vi "Write session and device.vi"(8 "error in (no error)":errorcluster, 9 "SLSC Device":refnum<k21>, 10 "SLSC Session in":refnum<class "SLSC Interface.lvclass">, 11 "SLSC Switch in":refnum<class "SLSC Switch.lvclass">) -> (0 "error out":errorcluster, 3 "SLSC Switch out":refnum<class "SLSC Switch.lvclass">)   [LabVIEW 2015, in "SLSC Switch.lvlib" / "SLSC Switch.lvclass"]
uses:
  SLSC Switch.lvclass
  <vilib>/National Instruments/SLSC Local or Remote Interface/SLSC Interface Class/SLSC Interface.lvclass
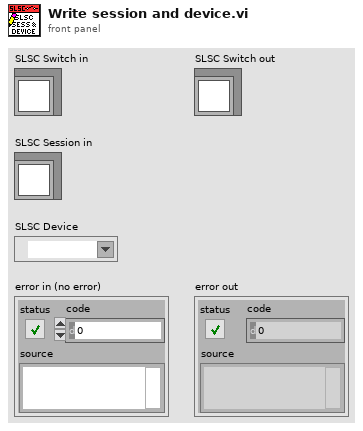
[diagram p1: front panel]
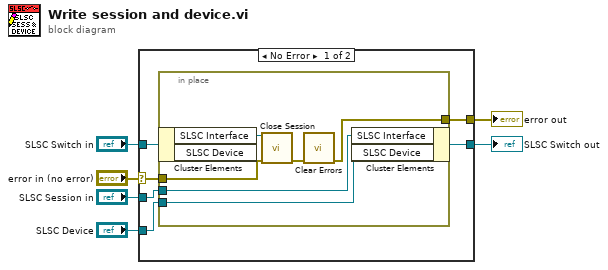
[diagram p0: block diagram]
diagram:
  n1 = case shown="No Error" "error in (no error)" {
    selector: "error in (no error)" -> [w10 w19]
    tunnel: "SLSC Switch in" -> [w12 w20]
    tunnel: [w11 w20] -> w5
    tunnel: [w9 w19] -> w3
    tunnel: "SLSC Device" -> [w8 _]
    tunnel: "SLSC Session in" -> [w7 _]
    frame No Error {
      n2 = in-place {
        in-place-border: w10 -> [w14]
        in-place-border: [w18] -> w9
        in-place-border: w8 -> [w17]
        in-place-border: w7 -> [w16]
        n3 = in-place-cluster #1(w12) -> ("SLSC Interface"=w15:refnum<class "SLSC Interface.lvclass">)  [unwired: 1 out]
        n4 = call-dynamic "Close Session.vi"("SLSC Interface in"=w15, "error in (no error)"=w14) -> ("error out"=w13:errorcluster)  [unwired: 13 in]
        n5 = call <vilib>:"Clear Errors.vi"("error in (no error)"=w13) -> ("error out"=w18:errorcluster)  [unwired: 5 in, 1 out]
        n6 = in-place-cluster #1("SLSC Interface"=w16, "SLSC Device"=w17) -> (w11:refnum<class "SLSC Switch.lvclass">)
      }
    }
    frame Error {
    }
  }
  "SLSC Switch out" <- w5
  "error out" <- w3
